vi "mtsToUt100ms.vi"(11 "m/s":dbl) -> (3 "u/100ms":dbl)   [LabVIEW 2019]
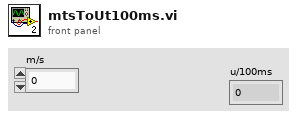
[diagram p1: front panel]
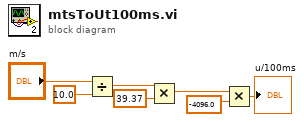
[diagram p0: block diagram]
diagram:
  n1 = Divide(x="m/s", y=10.0) -> (x/y=w6:dbl)
  n2 = Multiply(x=w6, y=39.37) -> (x*y=w4:dbl)
  n3 = Multiply(x=w4, y=-4096.0) -> (x*y=→"u/100ms":dbl)
